vi "Parse Path Component.vi"(10 "Pct-Encode (F)":bool, 11 "path":string) -> (2 "valid":bool, 3 "Segments":string[](array[string]))   [LabVIEW 2013, in "openURI.lvlib"]
uses:
  openURI.lvlib
  components/path/URI-Component.Path.lvclass/URI-Component.Path.ctl
  Percent-Decode String.vi
  isHEXDigit.vi
  components/path/URI-Component.Path.lvclass
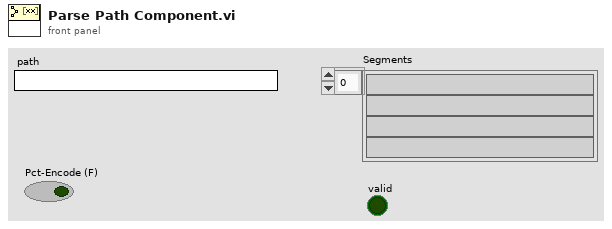
[diagram p1: front panel]
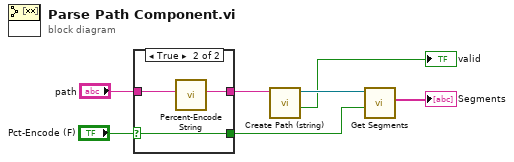
[diagram p0: block diagram]
diagram:
  n1 = case shown="True" "Pct-Encode (F)" {
    selector: "Pct-Encode (F)" -> [w8 w10]
    tunnel: "path" -> [w9 w12]
    tunnel: [w9 w11] -> w3
    tunnel: [w8 w10] -> w1
    frame False {
    }
    frame True {
      n2 = call "Percent-Encode String.vi"("String"=w12) -> ("Pct-Encoded String"=w11:string)  [unwired: 10 in]
    }
  }
  n3 = call "Create Path (string).vi"("Path"=w3) -> ("Valid"=→"valid":bool, "URI-Component.Path"=w7:refnum<class "URI-Component.Path.lvclass">)  [unwired: 7 in, 2 out]
  n4 = call "Get Segments.vi"("Pct-Encoded? (F)"=w1, "URI-Component.Path in"=w7) -> ("Segments"=→"Segments":string[])  [unwired: 7 in, 2 out]
